vi "temp_measure.vi"() -> ()   [LabVIEW 2019]
uses:
  <vilib>/DAQmx/read.llb/DAQmx Read (Analog 2D DBL NChan NSamp).vi
  <vilib>/DAQmx/read.llb/DAQmx Read (Analog DBL 1Chan 1Samp).vi
  <vilib>/DAQmx/miscellaneous.llb/DAQmx Fill In Error Info.vi
panel:
  out "Waveform Graph":dbl[][](graph)
  out "Array":dbl[][](array[slide]) scale=0.0..100.0
  out "Thermometer":dbl(slide) scale=0.0..100.0
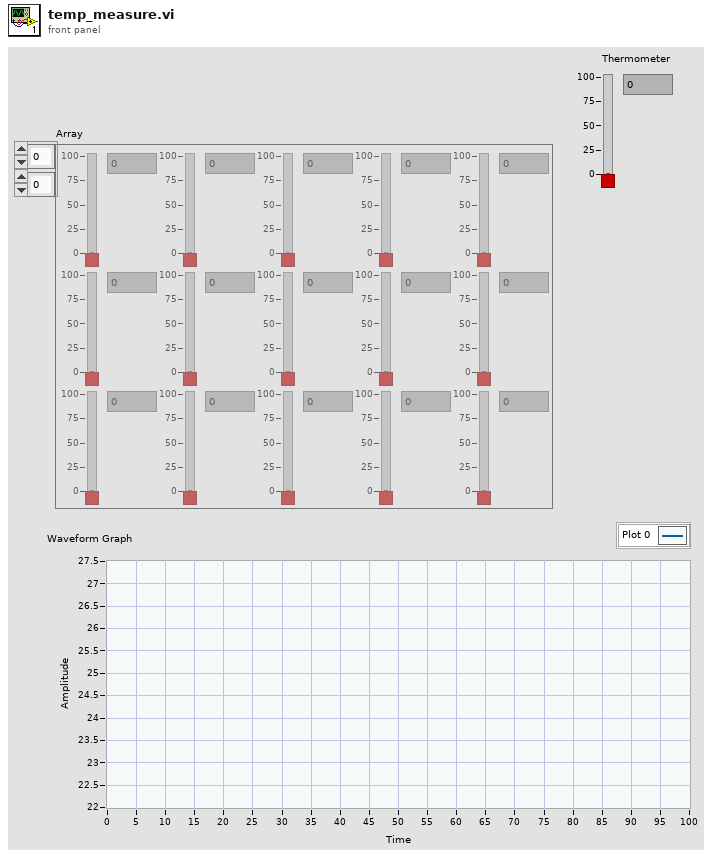
[diagram p1: front panel]
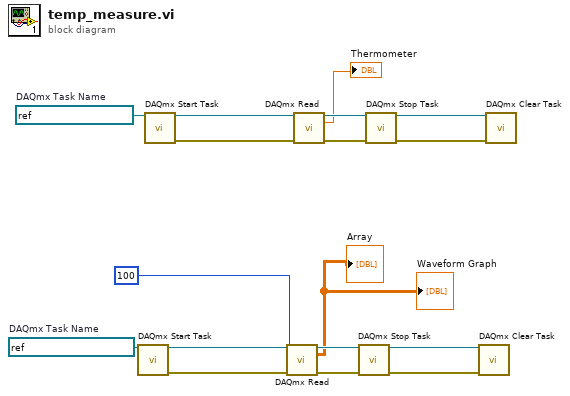
[diagram p0: block diagram]
diagram:
  w9 = refnum<k21> "3channel_nsample"  # DAQmx Task Name
  w11 = refnum<k21> "TemperatureTask"  # DAQmx Task Name
  n1 = call <vilib>:"DAQmx Start Task.vi"("task/channels in"=w9) -> ("task out"=w3:refnum<k21>, "error out"=w6:errorcluster)  [unwired: 13 in]
  n2 = call <vilib>:"DAQmx Start Task.vi"("task/channels in"=w11) -> ("task out"=w17:refnum<k21>, "error out"=w14:errorcluster)  [unwired: 13 in]
  n3 = call-poly <vilib>:"DAQmx Read.vi"("task/channels in"=w3, "number of samples per channel"=100, "error in"=w6) -> ("task out"=w4:refnum<k21>, "data"=→"Array" →"Waveform Graph":dbl[][], "error out"=w7:errorcluster)  [unwired: 10 in]
  n4 = call-poly <vilib>:"DAQmx Read.vi"("task/channels in"=w17, "error in"=w14) -> ("task out"=w16:refnum<k21>, "data"=→"Thermometer":dbl, "error out"=w13:errorcluster)  [unwired: 11 in]
  n5 = call <vilib>:"DAQmx Stop Task.vi"("task/channels in"=w4, "error in"=w7) -> ("task out"=w5:refnum<k21>, "error out"=w8:errorcluster)  [unwired: 12 in]
  n6 = call <vilib>:"DAQmx Stop Task.vi"("task/channels in"=w16, "error in"=w13) -> ("task out"=w15:refnum<k21>, "error out"=w12:errorcluster)  [unwired: 12 in]
  n7 = call <vilib>:"DAQmx Clear Task.vi"("task in"=w5, "error in"=w8) -> ()  [unwired: 13 in, 1 out]
  n8 = call <vilib>:"DAQmx Clear Task.vi"("task in"=w15, "error in"=w12) -> ()  [unwired: 13 in, 1 out]
